vi "LookUpTable.vi"(8 "Allowable Error in Distance":dbl, 9 "Speeds":dbl[](array[numeric])=[0.0, 0.0], 10 "Distances":dbl[](array[numeric])=[0.0, 1.0], 11 "Required Distance":dbl) -> (2 "Allowable Error in Wheel Speed":dbl, 3 "Required Speed":dbl)   [LabVIEW 2012]
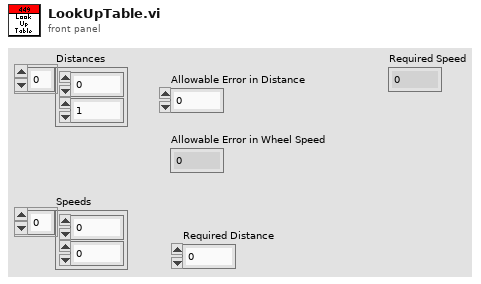
[diagram p1: front panel]
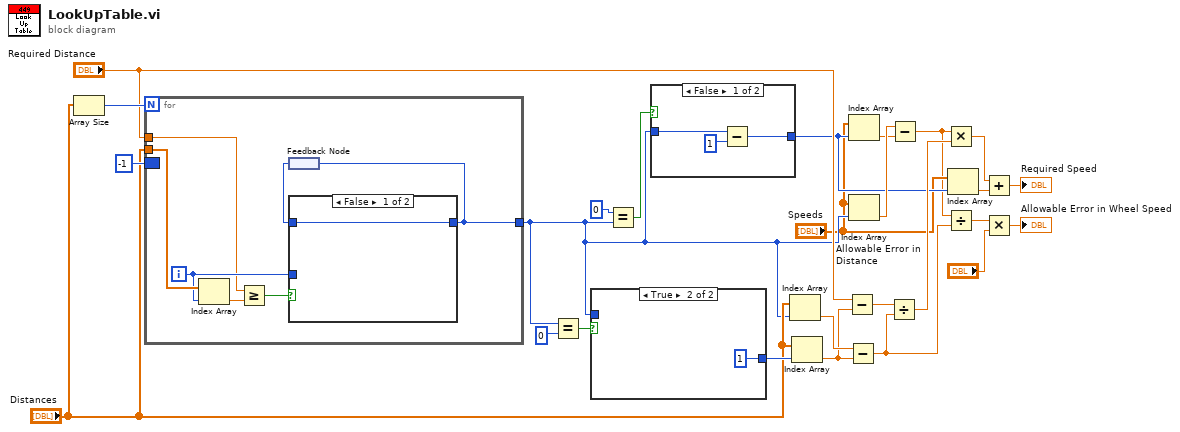
[diagram p0: block diagram]
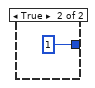
[diagram p2: hidden frame]
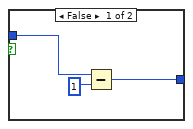
[diagram p3: hidden frame]
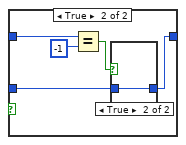
[diagram p4: hidden frame]
diagram:
  n1 = Array Size(array="Distances") -> (size(s)=w26:i32)
  n2 = for {
    N: w26 -> [_]
    tunnel: "Required Distance" -> [w28]
    tunnel: "Distances" -> [w33]
    border: -1 -> [_]
    tunnel: [w30] -> w15
    i -> [w32]
    n3 = Index Array(array=w33, index=w32) -> (element=w27:dbl)
    n4 = Greater Or Equal?(x=w28, y=w27) -> (x >= y?=w29:bool)
    n5 = feedback #1() -> (w31:i32)
    n6 = case shown="False" w29 {
      tunnel: w31 -> [w34 w39]
      tunnel: w32 -> [_ w36]
      tunnel: [w34 w35] -> w30
      frame False {
      }
      frame True {
        n7 = Equal?(x=w39, y=-1) -> (x = y?=w37:bool)
        n8 = case shown="True" w37 {
          tunnel: [w40 w41] -> w35
          tunnel: w36 -> [w40 w41]
          frame False {
          }
          frame True {
          }
        }
      }
    }
    n9 = feedback-in #1(w30) -> ()
  }
  n10 = Equal?(x=w15, y=0) -> (x = y?=w22:bool)
  n11 = case shown="True" w22 {
    tunnel: [w42 1 ("y")] -> w21
    tunnel: w15 -> [w43 _]
    frame False {
      n12 = Subtract(x=w43, y=1) -> (x-y=w42:i32)
    }
    frame True {
    }
  }
  n13 = Equal?(x=0, y=w15) -> (x = y?=w16:bool)
  n14 = case shown="False" w16 {
    tunnel: [w46 1] -> w11
    tunnel: w15 -> [w48 _]
    frame False {
      n15 = Subtract(x=w48, y=1) -> (x-y=w46:i32)
    }
    frame True {
    }
  }
  n16 = Index Array(array="Distances", index=w15) -> (element=w3:dbl)
  n17 = Index Array(array="Distances", index=w21) -> (element=w2:dbl)
  n18 = Subtract(x="Required Distance", y=w2) -> (x-y=w7:dbl)
  n19 = Subtract(x=w3, y=w2) -> (x-y=w1:dbl)
  n20 = Index Array(array="Speeds", index=w11) -> (element=w9:dbl)
  n21 = Index Array(array="Speeds", index=w15) -> (element=w12:dbl)
  n22 = Divide(x=w7, y=w1) -> (x/y=w19:dbl)
  n23 = Subtract(x=w12, y=w9) -> (x-y=w8:dbl)
  n24 = Multiply(x=w8, y=w19) -> (x*y=w18:dbl)
  n25 = Divide(x=w8, y=w1) -> (x/y=w6:dbl)
  n26 = Index Array(array="Speeds", index=w11) -> (element=w14:dbl)
  n27 = Add(x=w18, y=w14) -> (x+y=→"Required Speed":dbl)
  n28 = Multiply(x=w6, y="Allowable Error in Distance") -> (x*y=→"Allowable Error in Wheel Speed":dbl)
